vi "Read Numeric as CEXT.vi"(8 "error in (no error)":errorcluster, 10 "Tag":string, 11 "Var Bus in":refnum<class "Omni_Bus.lvclass">) -> (0 "error out":errorcluster, 2 "Numeric":cxt, 3 "Var Bus out":refnum<class "Omni_Bus.lvclass">)   [LabVIEW 2021, in "Omni_Bus.lvclass"]
uses:
  Omni_Bus.lvclass
  Omni_Bus.lvclass/Omni_Bus.ctl
  <vilib>/TSA/Abstract Data Classes/Abs_Types/Numeric/Abs_Numeric.lvclass
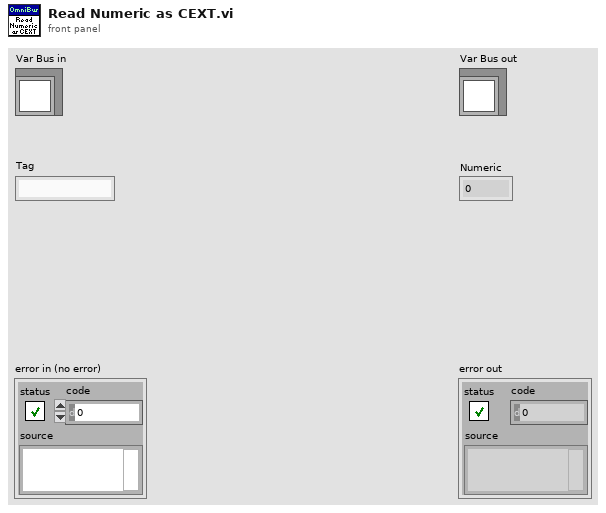
[diagram p1: front panel]
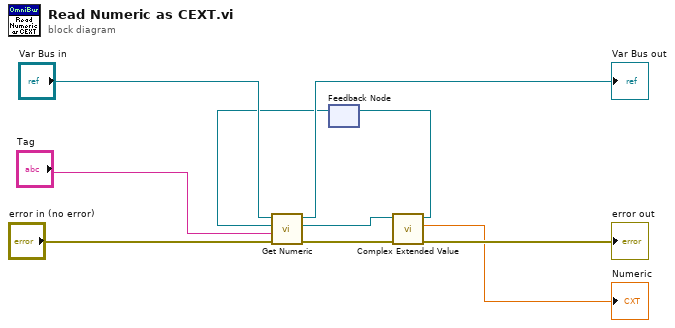
[diagram p0: block diagram]
diagram:
  n1 = feedback #1() -> (w1:refnum<class "Abs_Numeric.lvclass">)  [unwired: 1 in]
  n2 = call-dynamic "Get Numeric.vi"("error in (no error)"="error in (no error)", "Tag"="Tag", "Value Type"=w1, "Var Bus in"="Var Bus in") -> ("error out"=w3:errorcluster, "Value Out"=w2:refnum<class "Abs_Numeric.lvclass">, "Var Bus out"=→"Var Bus out":refnum<class "Omni_Bus.lvclass">)  [unwired: 5 in]
  n3 = call-dynamic "Complex Extended Value.vi"("error in (no error)"=w3, "Numeric in"=w2) -> ("error out"=→"error out":errorcluster, "Complex Double Float"=→"Numeric":cxt, "Numeric out"=w4:refnum<class "Abs_Numeric.lvclass">)  [unwired: 7 in]
  n4 = feedback-in #1(w4) -> ()
